vi "Get Version from EXE.vi"(0 "EXE Name":string, 11 "error in (no error)":errorcluster) -> (4 "Name and Version":string, 6 "Version":i32, 15 "error out":errorcluster)   [LabVIEW 2013]
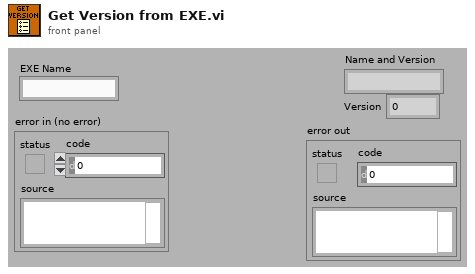
[diagram p1: front panel]
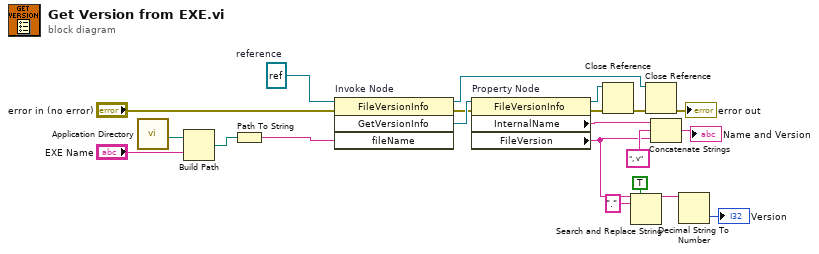
[diagram p0: block diagram]
diagram:
  w21 = refnum<k24> refnum  # reference
  n1 = call <vilib>:"Application Directory.vi"() -> ("Application Directory"=w3:path)
  n2 = Build Path(base path=w3, name or relative path="EXE Name") -> (appended path=w1:path)
  n3 = Path To String(path=w1) -> (string=w20:string)
  n4 = invoke on="Invoke Node" class="FileVersionInfo" method="GetVersionInfo"(reference=w21, error in="error in (no error)", "fileName"=w20) -> (reference out=w14:refnum<k24>, error out=w18:errorcluster, "GetVersionInfo"=w19:refnum<k24>)  [unwired: 1 in, 1 out]
  n5 = property on="Property Node" class="FileVersionInfo"(reference=w19, error in=w18) -> (reference out=w17:refnum<k24>, error out=w16:errorcluster, "InternalName"=w13:string, "FileVersion"=w8:string)
  n6 = Close Reference(reference=w17, error in (no error)=w16) -> (error out=w15:errorcluster)
  n7 = Search and Replace String(replace all?=TRUE ("replace all? (F)"), input string=w8, search string=".") -> (result string=w5:string)  [unwired: 5 in, 3 out]
  n8 = Close Reference(reference=w14, error in (no error)=w15) -> (error out=→"error out":errorcluster)
  n9 = Concatenate Strings(w13, ", v" ("string"), w8) -> (→"Name and Version":string)
  n10 = Decimal String To Number(string=w5) -> (number=→"Version":i32)  [unwired: 2 in, 1 out]
